vi "test - Read CSM File Logger Config.vi"(8 "error in (no error)":errorcluster, 11 "TestCase in":refnum<class "csm-ini-variable-addon.lvclass">) -> (0 "error out":errorcluster, 3 "TestCase out":refnum<class "csm-ini-variable-addon.lvclass">)   [LabVIEW 2017, in "csm-ini-variable-addon.lvclass"]
uses:
  csm-ini-variable-addon.lvclass
  <vilib>/addons/_JKI Toolkits/VI Tester/TestCase.llb/TestCase.lvclass
  INI-Static-Variable-Support/LabVIEW-Config/LabVIEW-Config.lvlib
  INI-Static-Variable-Support/INI-Static-Variable-Support.lvlib
  C:/Program Files (x86)/National Instruments/LabVIEW 2017/vi.lib/addons/_JKI Toolkits/VI Tester/TestCase.llb/TestCase.lvclass
panel:
  out "FileLogger Configuration-v1":T1={"Enable"=TRUE, "Limit"={"FileSize"=10000000, "FileNum"=2}, "Timestamp.Format"="%<%Y/%m/%d %H:%M:%S%3u>T", "AutoExit"=FALSE} {"Limit"."FileSize" format="%.0p"}
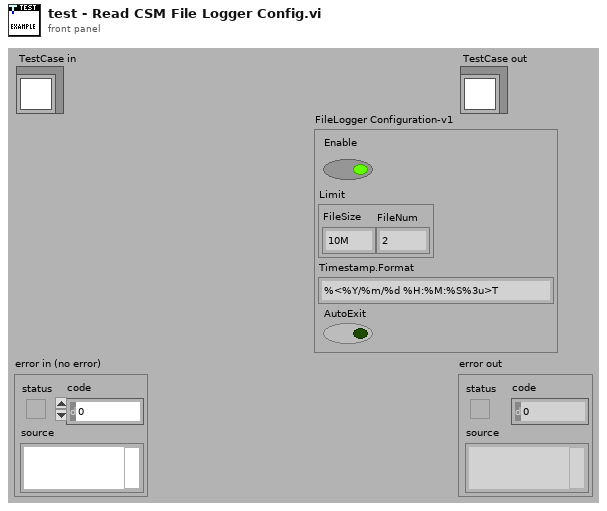
[diagram p1: front panel]
types:
  T1 = cluster{"Enable":bool, "Limit":cluster{"FileSize":i64, "FileNum":i32}, "Timestamp.Format":string, "AutoExit":bool}
  T2 = typedef "LabVIEW-Config.lvlib/Config.ctl" = cluster{"Path":path, "Lines":string[], "Tokens":T3[], "Modified?":bool}
  T3 = typedef "LabVIEW-Config.lvlib/LineToken.ctl" = enum8{"comment", "section", "key", "more"}
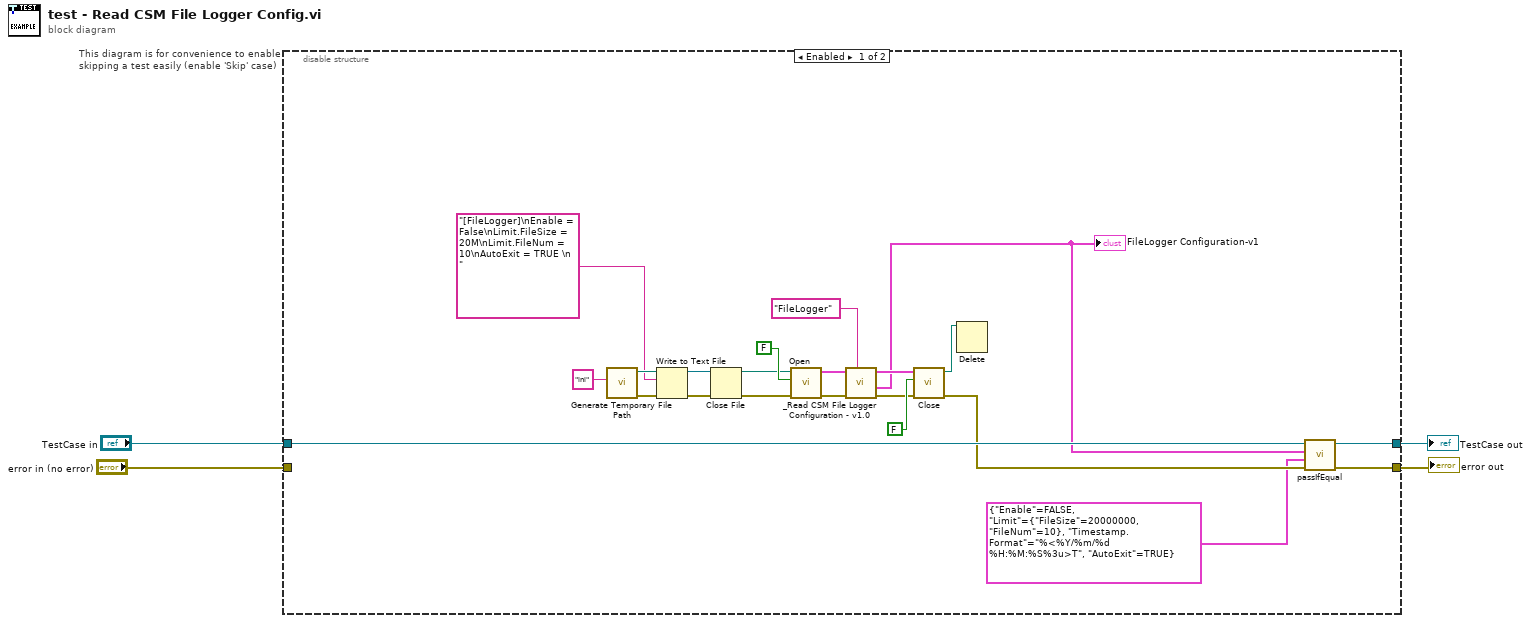
[diagram p0: block diagram]
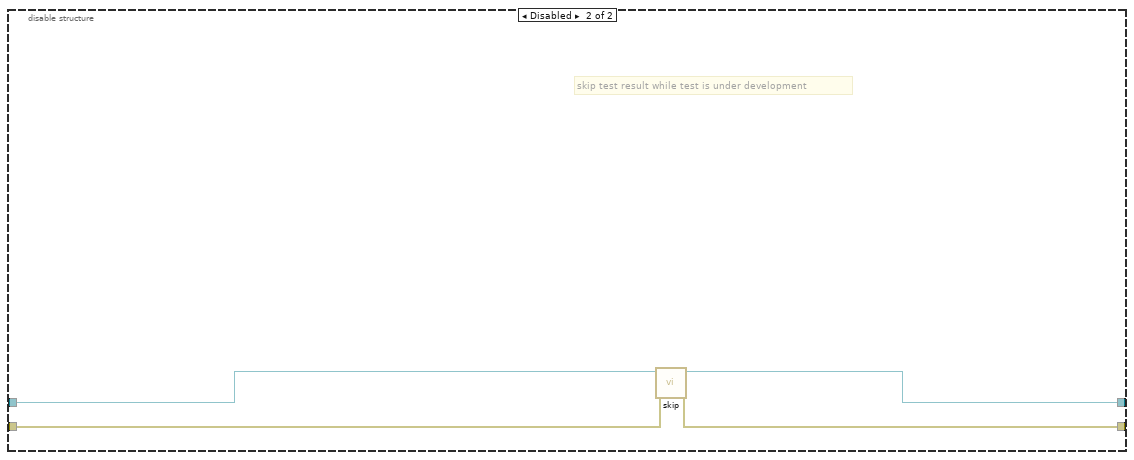
[diagram p2: hidden frame]
diagram:
  n1 = disable-structure "This diagram is for convenience to enable skipping a test easily (enable 'Skip' case)" shown="Enabled" {
    disable-tunnel: "TestCase in" -> [w26 w30]
    disable-tunnel: [w25 w28] -> w1
    disable-tunnel: [w24 w29] -> w3
    disable-tunnel: "error in (no error)" -> [_ w27]
    frame Enabled {
      # "Create temporary ini file"
      n2 = call <vilib>:"Generate Temporary File Path.vi"("Temporary File Extension (tmp)"="ini") -> ("error out"=w21:errorcluster, "Unique Temporary File Path"=w18:path)  [unwired: 9 in]
      n3 = Write to Text File(file (use dialog)=w18, text="[FileLogger]\nEnable = False\nLimit.FileSize = 20M\nLimit.FileNum = 10\nAutoExit = TRUE \n ", error in=w21) -> (refnum out=w17:refnum<file>, error out=w19:errorcluster)  [unwired: 1 in, 1 out]
      n4 = Close File(refnum=w17, error in=w19) -> (path=w13:path, error out=w14:errorcluster)
      n5 = call "Open.vi"("error in (no error)"=w14, "Create if not exists? (T)"=FALSE, "Path"=w13) -> ("error out"=w12:errorcluster, "Config"=w10:T2)  [unwired: 5 in, 2 out]
      n6 = call "_Read CSM File Logger Configuration - v1.0.vi"("Section Name"="FileLogger", "error in (no error)"=w12, "Config"=w10) -> ("error out"=w11:errorcluster, "FileLogger Configuration-v1"=w6:T1, "Config out"=w9:T2)  [unwired: 6 in]
      "FileLogger Configuration-v1" <- w6
      n7 = call "Close.vi"("error in (no error)"=w11, "Write if modified? (T)"=FALSE, "Config"=w9) -> ("error out"=w8:errorcluster, "Path"=w15:path)  [unwired: 7 in]
      n8 = Delete(path (use dialog)=w15) -> ()  [unwired: 4 in, 3 out]
      n9 = call-dynamic "passIfEqual.vi"("error in (no error)"=w8, "y"=T1 {"Enable"=FALSE, "Limit"={"FileSize"=20000000, "FileNum"=10}, "Timestamp.Format"="%<%Y/%m/%d %H:%M:%S%3u>T", "AutoExit"=TRUE} ("FileLogger Configuration-v1"), "x"=w6, "TestCase in"=w26) -> ("error out"=w24:errorcluster, "TestCase out"=w25:refnum<class "csm-ini-variable-addon.lvclass">)  [unwired: 6 in]
    }
    frame Disabled {
      # "skip test result while test is under development"
      n10 = call <vilib>:"skip.vi"("error in (no error)"=w27, "TestCase in"=w30) -> ("error out"=w29:errorcluster, "TestCase out"=w28:refnum<class "csm-ini-variable-addon.lvclass">)  [unwired: 8 in]
    }
  }
  "error out" <- w3
  "TestCase out" <- w1
